vi "Begin Transfer.vi"(8 "error in":errorcluster, 9 "Retry Delay":i32 format="%d ms", 10 "SDO Transfer in":refnum<class "SDO Transfer.lvclass">, 11 "SDO Manager":refnum<class "SDO Manager.lvclass">) -> (0 "error out":errorcluster)   [LabVIEW 2020, in "CANopen.lvlib" / "SDO Manager.lvlib" / "SDO Manager.lvclass"]
uses:
  SDO Manager.lvclass
  SDO Transfer/SDO Transfer.lvclass
  SDO Transfer/SDO Transfer.lvclass/SDO Transfer.ctl
  SDO Manager.lvclass/SDO Manager.ctl
  Transfer Beginner Messages/Begin Transfer Msg/Begin Transfer Msg.lvclass/Begin Transfer Msg.ctl
  <vilib>/ActorFramework/Message Enqueuer/Message Enqueuer.lvclass/Message Enqueuer.ctl
  Transfer Beginner/Transfer Beginner.lvclass
  C:/Program Files/National Instruments/LabVIEW 2026/vi.lib/ActorFramework/Actor/Actor.lvclass
  Transfer Beginner/Transfer Beginner.lvclass/Transfer Beginner.ctl
  Transfer Beginner/Set Max Retries.vi
  Transfer Beginner/Set Retry Delay.vi
  <vilib>/ActorFramework/Message Enqueuer/Enqueue.vi
  Transfer Beginner Messages/Begin Transfer Msg/Begin Transfer Msg.lvclass
  C:/Program Files/National Instruments/LabVIEW 2026/vi.lib/ActorFramework/Message/Message.lvclass
  <vilib>/Utility/LVClass/Get LV Class Name.vi
  <vilib>/ActorFramework/tracing/Trace Generation/Generate Trace for Message.vi
  <vilib>/ActorFramework/Message Priority Queue/Priority Enqueue.vi
  <vilib>/ActorFramework/Actor/Actor.lvclass
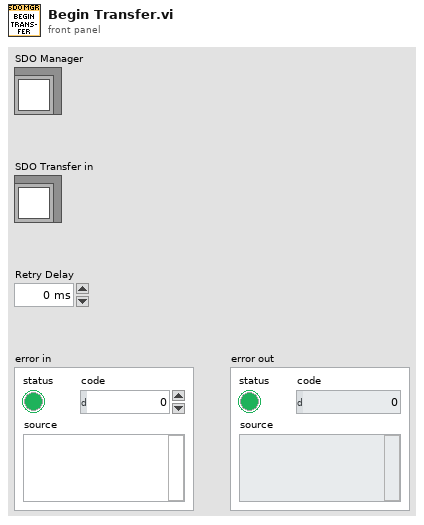
[diagram p1: front panel]
types:
  T1 = map{u8, refnum<class "Message Enqueuer.lvclass">}
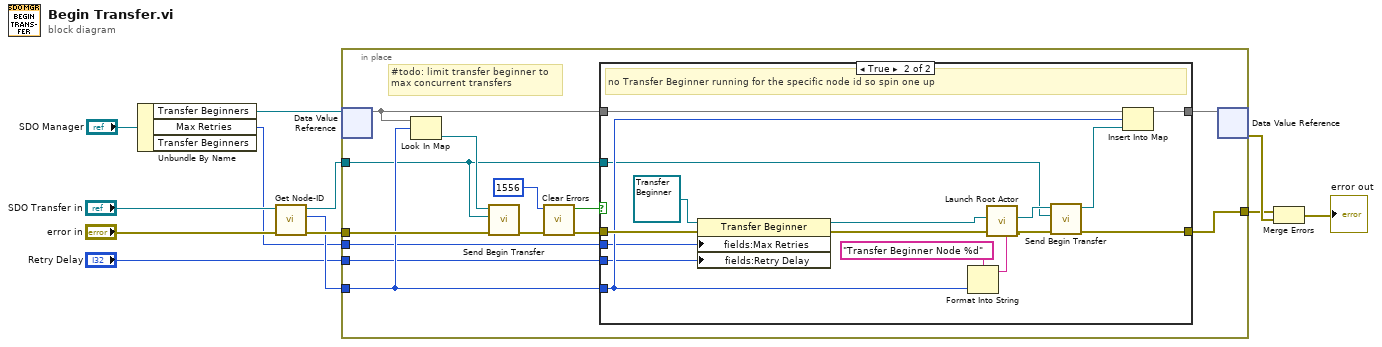
[diagram p0: block diagram]
diagram:
  n1 = Unbundle By Name("SDO Manager") -> ("Transfer Beginners"=w3:refnum<data-value>, "Max Retries"=w2:u8)  [unwired: 1 out]
  n2 = call "Get Node-ID.vi"("error in"="error in", "SDO Transfer in"="SDO Transfer in") -> ("error out"=w8:errorcluster, "Node-ID"=w5:u8, "SDO Transfer out"=w6:refnum<class "SDO Transfer.lvclass">)  [unwired: 7 in]
  n3 = in-place {
    in-place-border: w5 -> [w20]
    in-place-border: w6 -> [w13]
    in-place-border: w8 -> [w24]
    in-place-border: [w23] -> w10
    in-place-border: w2 -> [w18]
    in-place-border: "Retry Delay" -> [w17]
    # "#todo: limit transfer beginner to\nmax concurrent transfers"
    n4 = in-place-dvr #1(w3) -> (w21:T1)  [unwired: 1 out]
    n5 = Look In Map(map=w21, key=w20) -> (value=w25:refnum<class "Message Enqueuer.lvclass">)  [unwired: 1 in, 1 out]
    n6 = call "Send Begin Transfer.vi"("error in (no error)"=w24, "SDO Transfer"=w13, "Message Enqueuer"=w25) -> ("error out"=w22:errorcluster)  [unwired: 7 in, 1 out]
    n7 = call <vilib>:"Clear Errors.vi"("error in (no error)"=w22, "specific error code to clear (0: all)"=1556) -> ("error out"=w16:errorcluster, "specific error cleared?"=w14:bool)  [unwired: 4 in]
    n8 = case shown="True" w14 {
      tunnel: [w27 w31] -> w23
      tunnel: w21 -> [w26 w41]
      tunnel: w20 -> [_ w37]
      tunnel: [w26 w40] -> w19
      tunnel: w18 -> [_ w33]
      tunnel: w17 -> [_ w32]
      tunnel: w16 -> [w27 w43]
      tunnel: w13 -> [_ w28]
      frame False {
        # "Transfer Beginner for that specific channel running"
      }
      frame True {
        # "no Transfer Beginner running for the specific node id so spin one up"
        n9 = property class="Transfer Beginner"(reference=refnum<class "Transfer Beginner.lvclass"> refnum ("CANopen.lvlib:Transfer Beginner.lvlib:Transfer Beginner.lvclass"), error in=w43, "fields:Max Retries"=w33, "fields:Retry Delay"=w32) -> (reference out=w34:refnum<class "Transfer Beginner.lvclass">, error out=w36:errorcluster)
        n10 = Format Into String(format string="Transfer Beginner Node %d" ("Debug Alias"), w37) -> (resulting string=w39:string)  [unwired: 2 in, 1 out]
        n11 = call <vilib>:"Launch Root Actor.vi"("Debug Alias"=w39, "error in (no error)"=w36, "Actor"=w34) -> ("error out"=w42:errorcluster, "Actor's Enqueuer"=w30:refnum<class "Message Enqueuer.lvclass">)  [unwired: 7 in]
        n12 = call "Send Begin Transfer.vi"("error in (no error)"=w42, "SDO Transfer"=w28, "Message Enqueuer"=w30) -> ("error out"=w31:errorcluster, "Message Enqueuer out"=w29:refnum<class "Message Enqueuer.lvclass">)  [unwired: 7 in]
        n13 = Insert Into Map(map in=w41, key=w37, value=w29) -> (map out=w40:T1)  [unwired: 2 out]
      }
    }
    n14 = in-place-dvr #1(w19) -> (w11:errorcluster)  [unwired: 1 out]
  }
  n15 = Merge Errors(w10, w11) -> (→"error out":errorcluster)
